vi "Rcv Cmd.vi"(8 "error in":errorcluster, 11 "Instrument in":refnum<class "Instrument.lvclass">) -> (0 "error out":errorcluster, 3 "Instrument out":refnum<class "Instrument.lvclass">)   [LabVIEW 2017, in "Instrument.lvclass"]
uses:
  Instrument.lvclass
  Instrument.lvclass/Instrument.ctl
  state.ctl
  Command/Command.lvclass
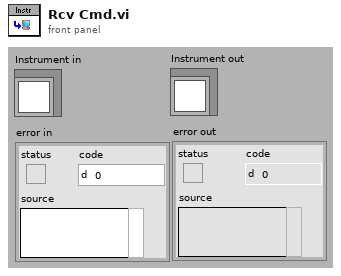
[diagram p1: front panel]
types:
  T1 = typedef "Instrument.lvclass/state.ctl" = enum8{"Configure", "Acquire", "Wait", "Quit", "Handle Error", "NOOP"}
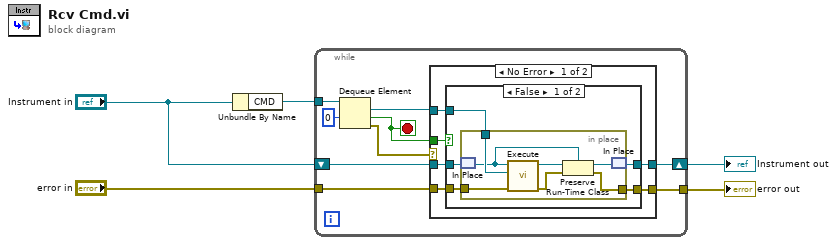
[diagram p0: block diagram]
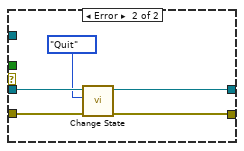
[diagram p3: hidden frame]
diagram:
  n1 = Unbundle By Name("Instrument in") -> ("CMD"=w5:refnum<queue>)
  n2 = while {
    tunnel: w5 -> [w14]
    tunnel: [w10] -> w2
    tunnel: "error in" -> [w9]
    shift-right: [w12] -> w1
    shift-left: "Instrument in" -> [w13]
    stop <- w8 stop-if-true
    n3 = Dequeue Element(queue=w14, timeout in ms (-1)=0) -> (element=w11:refnum<class "Command.lvclass">, timed out?=w8:bool, error out=w7:errorcluster)  [unwired: 1 in, 1 out]
    n4 = case shown="No Error" w7 {
      tunnel: w13 -> [w20 w39]
      tunnel: [w19 w38] -> w12
      tunnel: w11 -> [w18 _]
      tunnel: [w17 w37] -> w10
      tunnel: w9 -> [w16 w36]
      tunnel: w8 -> [w15 _]
      frame No Error {
        n5 = case shown="False" w15 {
          tunnel: w20 -> [w25 w33]
          tunnel: [w24 w33] -> w19
          tunnel: w18 -> [w23 _]
          tunnel: [w22 w34] -> w17
          tunnel: w16 -> [w21 w34]
          frame False {
            n6 = in-place {
              in-place-border: w23 -> [w32]
              in-place-border: [w28] -> w22
              in-place-border: w21 -> [w27]
              n7 = in-place-match #1(w25) -> (w26:refnum<class "Instrument.lvclass">)
              n8 = call "Execute.vi"("error in"=w27, "Command in"=w32, "Object In"=w26) -> ("error out"=w29:errorcluster, "Object Out"=w31:refnum<class>)  [unwired: 7 in]
              n9 = Preserve Run-Time Class(object in=w31, error in=w29, 2:w26) -> (object out=w30:refnum<class "Instrument.lvclass">, error out=w28:errorcluster)
              n10 = in-place-match #1(w30) -> (w24:refnum<class "Instrument.lvclass">)
            }
          }
          frame True {
          }
        }
      }
      frame Error {
        n11 = call "Change State.vi"("error in"=w36, "instr state"=state."Quit", "Instrument in"=w39) -> ("error out"=w37:errorcluster, "Instrument out"=w38:refnum<class "Instrument.lvclass">)  [unwired: 7 in]
      }
    }
  }
  "error out" <- w2
  "Instrument out" <- w1
